vi "AK Befehl Auswerten.vi"(10 "Array":string[](array[string])) -> (2 "String für schreiben":string)   [LabVIEW 2020, in "AK-Schnittstelle.lvlib"]
uses:
  AK-Schnittstelle.lvlib
  Aktionen Stoernummern pruefen.ctl
  Aktionen Zustandsfehlerinformation.ctl
  Funktionstasten/Zustaende.ctl
  Funktionstasten/Funktionstasten.lvlib
  Funktionstasten/Betriebsart.ctl
  Funktionstasten/Funktionstasten-Aktion.ctl
  Aktionen Gespeicherte Werte.ctl
  Seiten/Log Konfig/LogKonfig.lvlib
  Seiten/Log Konfig/Aktionen Trigger.ctl
  Seiten/FT-IR/FT-IR.lvlib
  Seiten/FT-IR/FGV FT-IR Gasliste Aktionen.ctl
  Messdaten/Messdaten.lvlib
  Messdaten/Aktionen FGV Messdaten.ctl
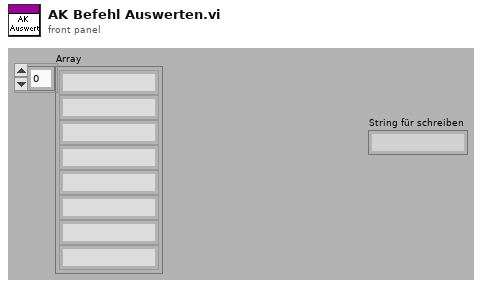
[diagram p1: front panel]
types:
  T1 = typedef "AK-Schnittstelle.lvlib/Aktionen Stoernummern pruefen.ctl" = enum16{"lesen", "prüfen"}
  T2 = typedef "AK-Schnittstelle.lvlib/Aktionen Zustandsfehlerinformation.ctl" = enum16{"OK", "Offline", "Busy", "Syntax Error", "Datenfehler"}
  T3 = typedef "AK-Schnittstelle.lvlib/Aktionen Gespeicherte Werte.ctl" = enum16{"lesen", "laden", "speichern", "Seriell", "TCP", "Diverse", "AKTIV", "AK-Namen"}
  T4 = typedef "Funktionstasten.lvlib/Funktionstasten-Aktion.ctl" = enum16{"Initialisieren", "Zustand setzen", "Taste gedrückt", "Fehler speichern", "Lesen", "Manuell", "Remote", "Bitparallel", "Samplepoint", "Zeit Prüfen", "reset Umschalten"}
  T5 = typedef "FT-IR.lvlib/FGV FT-IR Gasliste Aktionen.ctl" = enum16{"lesen", "Gasliste FT-IR", "Gasliste ausgelesen", "laden", "speichern", "löschen"}
  T6 = typedef "Messdaten.lvlib/Aktionen FGV Messdaten.ctl" = enum16{"lesen", "schreiben", "löschen", "Mittelwerte", "Komponente"}
  T7 = typedef "Funktionstasten.lvlib/Zustaende.ctl" = enum16{"Standby", "Pause", "Eco", "Messen", "Kalibrieren", "Spülen Filter", "Spülen Leitung", "Umgebungsluft", "0-Gas", "Cal-Gas", "CG zu PNS", "-------------", "Init 1", "Init 2", "Init 3", "Init 4", "Messen vorbereiten", "Messen durchführen", "Exit"}
  T8 = typedef "Funktionstasten.lvlib/Betriebsart.ctl" = enum16{"Manuell", "Remote", "Bitparallel"}
  T9 = typedef "LogKonfig.lvlib/Aktionen Trigger.ctl" = enum16{"lesen", "ALLE schreiben", "Trigger prüfen", "Trigger rücksetzen"}
  T10 = typedef "AK-Schnittstelle.lvlib/Diverse gespeicherte Werte.ctl" = cluster{"Kalibriergaseingang":i16, "SamplePoint":i16, "CalGas zu PNS":i16, "Gas-Reihenfolge":i16[], "Zeit 0-Gas":sgl, "Zeit CalGas":sgl, "AK Befehlssatz":T11}
  T11 = typedef "AK-Schnittstelle.lvlib/AK Befehlssatz.ctl" = enum16{"MEXA", "IAG v1.4", "AVL (Puma)", "PEUS"}
  T12 = typedef "LogKonfig.lvlib/Element Triggerereignisse.ctl" = cluster{"Trigger verwenden":T13, "Messwert":u16, "kl./gr.":u16, "Wert":sgl, "Puffergröße":sgl}
  T13 = typedef "LogKonfig.lvlib/Auswahlfeld aktiviert-deaktiviert.ctl" = u16
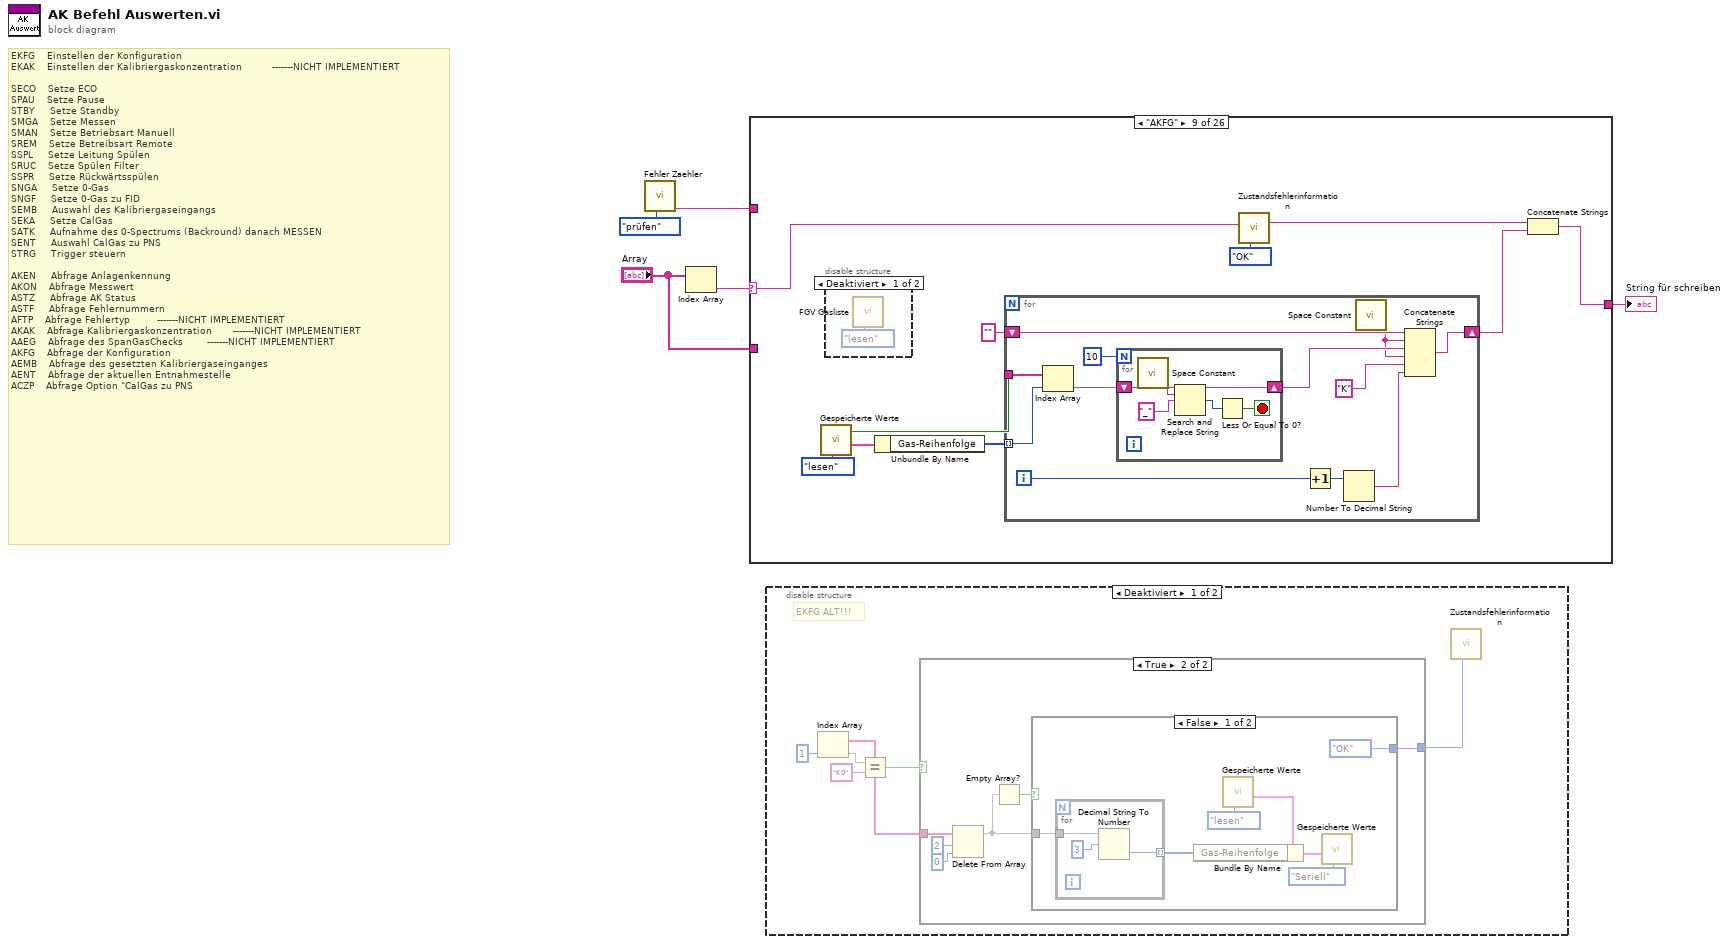
[diagram p0: block diagram]
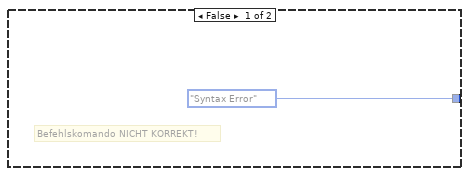
[diagram p2: hidden frame]
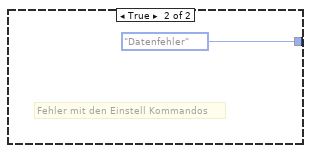
[diagram p3: hidden frame]
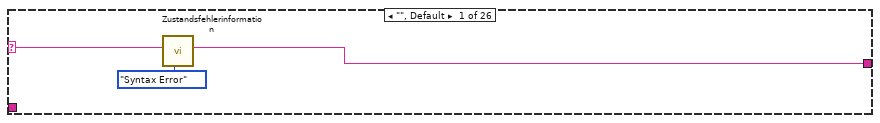
[diagram p5: hidden frame]
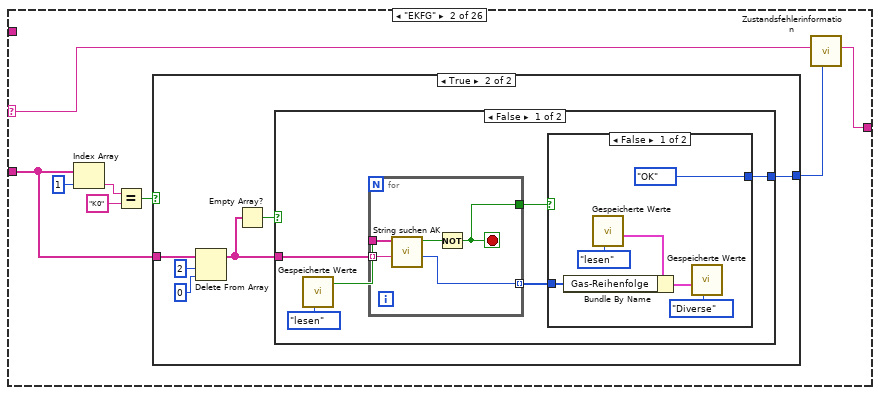
[diagram p6: hidden frame]
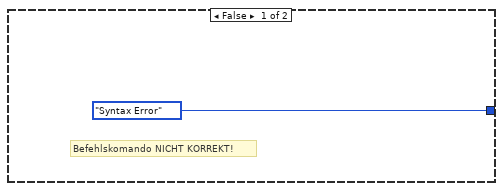
[diagram p7: hidden frame]
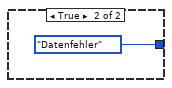
[diagram p8: hidden frame]
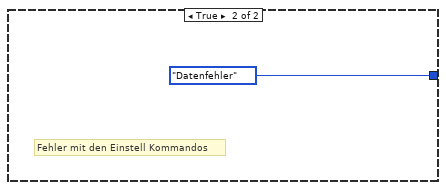
[diagram p9: hidden frame]
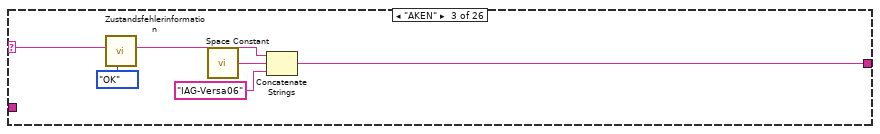
[diagram p10: hidden frame]
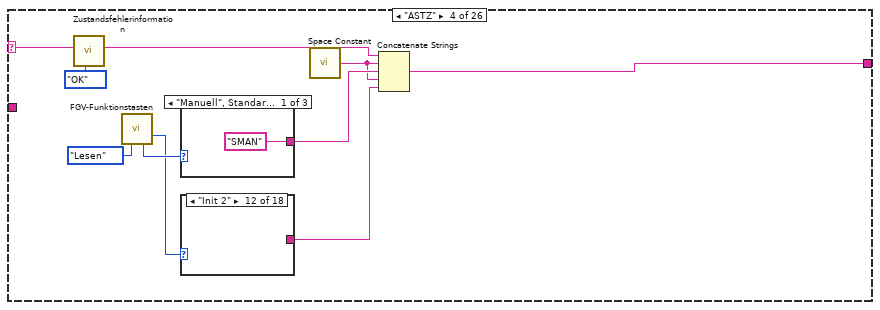
[diagram p11: hidden frame]
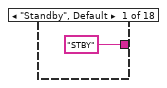
[diagram p12: hidden frame]
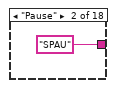
[diagram p13: hidden frame]
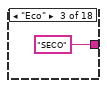
[diagram p14: hidden frame]
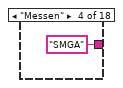
[diagram p15: hidden frame]
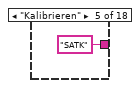
[diagram p16: hidden frame]
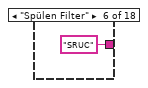
[diagram p17: hidden frame]
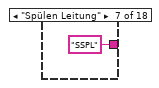
[diagram p18: hidden frame]
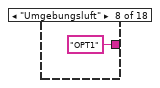
[diagram p19: hidden frame]
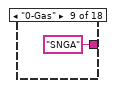
[diagram p20: hidden frame]
diagram:
  # "EKFG    Einstellen der Konfiguration\nEKAK    Einstellen der Kalibriergaskonzentration          -------NICHT IMPLEMENTIERT\n\nSECO    Setze ECO\nSPAU    Setze Pause\nSTBY     Setze Standby\nSMGA    Setze Messen\nSMAN    Setze Betriebsart Manuell\nSREM    Setze Betreibsart Remote\nSSPL     Setze Leitung Spülen\nSRUC    Setze Spülen Filter\nSSPR     Setze Rückwärtsspülen\nSNGA     Setze 0-Gas\nSNGF     Setze 0-Gas zu FID\nSEMB     Auswahl des Kalibriergaseingangs\nSEKA     Setze CalGas\nSATK     Aufnahme des 0-Spectrums (Backround) danach MESSEN\nSENT     Auswahl CalGas zu PNS\nSTRG     Trigger steuern\n\nAKEN     Abfrage Anlagenkennung\nAKON    Abfrage Messwert\nASTZ     Abfrage AK Status\nASTF     Abfrage Fehlernummern\nAFTP    Abfrage Fehlertyp         -------NICHT IMPLEMENTIERT\nAKAK    Abfrage Kalibriergaskonzentration       -------NICHT IMPLEMENTIERT\nAAEG    Abfrage des SpanGasChecks        -------NICHT IMPLEMENTIERT\nAKFG    Abfrage der Konfiguration\nAEMB    Abfrage des gesetzten Kalibriergaseinganges\nAENT    Abfrage der aktuellen Entnahmestelle\nACZP    Abfrage Option \"CalGas zu PNS"
  n1 = call "Fehler Zaehler.vi"("Aktionen"=Aktionen_Stoernummern_pruefen."prüfen") -> ("Fehlerzähler"=w3:string)  [unwired: 7 in, 3 out]
  n2 = Index Array(array="Array") -> (element=w2:string)  [unwired: 1 in]
  n3 = case shown="\"AKFG\"" w2 {
    selector: w2 -> [w7 w15 w45 w56 w76 w86 w95 w104 w114 w149 w194 w197 w200 w203 w206 w209 w213 w216 w220 w222 w235 w240 w261 w275 w279 w310]
    tunnel: [w6 w14 w47 w58 w78 w88 w97 w106 w116 w150 w193 w196 w199 w202 w205 w208 w212 w215 w219 w221 w234 w239 w260 w274 w278 w309] -> w5
    tunnel: w3 -> [_ _ _ _ _ _ _ _ _ _ _ _ _ _ _ _ _ _ _ _ _ _ _ _ _ _]
    tunnel: "Array" -> [_ w16 _ _ _ _ _ _ _ w140 _ _ _ _ _ _ _ _ _ _ _ w238 _ _ w277 w308]
    frame "", Default {
      n4 = call "Zustandsfehlerinformation.vi"("Aktionen"=Aktionen_Zustandsfehlerinformation."Syntax Error", "String"=w7) -> ("String"=w6:string)  [unwired: 9 in]
    }
    frame "EKFG" {
      n5 = Index Array(array=w16, index=1 ("Index")) -> (element=w12:string)
      n6 = Equal?(x=w12, y="K0") -> (x = y?=w10:bool)
      n7 = case shown="True" w10 {
        tunnel: w16 -> [_ w21]
        tunnel: [Aktionen_Zustandsfehlerinformation."Syntax Error" ("Aktionen") w18] -> w9
        frame False {
          # "Befehlskomando NICHT KORREKT!"
        }
        frame True {
          n8 = Delete From Array(array=w21, length=2 ("Länge"), index=0 ("Index")) -> (array with subset deleted=w20:string[])  [unwired: 1 out]
          n9 = Empty Array?(array=w20) -> (empty?=w19:bool)
          n10 = case shown="False" w19 {
            tunnel: w20 -> [w29 _]
            tunnel: [w25 Aktionen_Zustandsfehlerinformation."Datenfehler" ("Aktionen")] -> w18
            frame False {
              n11 = call "Gespeicherte Werte.vi"("Aktionen"=Aktionen_Gespeicherte_Werte."lesen") -> ("Port changed in"=w26:bool)  [unwired: 5 in, 5 out]
              n12 = for {
                tunnel: w29 -> [w32] mode=indexing
                tunnel: [w31] -> w28 mode=indexing
                tunnel: w26 -> [w33]
                tunnel: [w34] -> w24
                stop <- w34 stop-if-true
                n13 = call "String suchen AK.vi"("gesucht"=w32, "Namen"=w33) -> ("Index"=w31:i32, "Gefunden?"=w30:bool)  [unwired: 8 in]
                n14 = Not(x=w30) -> (.not. x?=w34:bool)
              }
              n15 = case shown="False" w24 {
                tunnel: w28 -> [w39 _]
                tunnel: [Aktionen_Zustandsfehlerinformation."OK" ("Aktionen") Aktionen_Zustandsfehlerinformation."Datenfehler" ("Aktionen")] -> w25
                frame False {
                  n16 = call "Gespeicherte Werte.vi"("Aktionen"=Aktionen_Gespeicherte_Werte."lesen") -> ("Diverse Werte"=w37:T10)  [unwired: 6 in, 4 out]
                  n17 = Bundle By Name(cluster=w37, "Gas-Reihenfolge"=w39) -> (w36:T10)
                  n18 = call "Gespeicherte Werte.vi"("Aktionen"=Aktionen_Gespeicherte_Werte."Diverse", "Diverse Werte"=w36) -> ()  [unwired: 5 in, 5 out]
                }
                frame True {
                }
              }
            }
            frame True {
              # "Fehler mit den Einstell Kommandos"
            }
          }
        }
      }
      n19 = call "Zustandsfehlerinformation.vi"("Aktionen"=w9, "String"=w15) -> ("String"=w14:string)  [unwired: 9 in]
    }
    frame "AKEN" {
      n20 = call "Zustandsfehlerinformation.vi"("Aktionen"=Aktionen_Zustandsfehlerinformation."OK", "String"=w45) -> ("String"=w44:string)  [unwired: 9 in]
      n21 = call <vilib>:"Space Constant.vi"() -> ("String"=w43:string)
      n22 = Concatenate Strings(w44, w43, "IAG-Versa06" ("String")) -> (w47:string)
    }
    frame "ASTZ" {
      n23 = call "Zustandsfehlerinformation.vi"("Aktionen"=Aktionen_Zustandsfehlerinformation."OK", "String"=w56) -> ("String"=w55:string)  [unwired: 9 in]
      n24 = call "FGV-Funktionstasten.vi"("Aktion"=Funktionstasten-Aktion."Lesen") -> ("ausgewählte Funktion"=w51:T7, "Betriebsart"=w53:T8)  [unwired: 7 in, 6 out]
      n25 = case shown="\"Manuell\", Standard" w53 {
        tunnel: ["SMAN" ("String") "SREM" ("String") "SBIT" ("String")] -> w52
        frame "Manuell", Default {
        }
        frame "Remote" {
        }
        frame "Bitparallel" {
        }
      }
      n26 = case shown="\"Init 2\"" w51 {
        tunnel: ["STBY" ("String") "SPAU" ("String") "SECO" ("String") "SMGA" ("String") "SATK" ("String") "SRUC" ("String") "SSPL" ("String") "OPT1" ("String") "SNGA" ("String") "OPT2" ("String") _ _ _ _ _ _ _ _] -> w49
        frame "Standby", Default {
        }
        frame "Pause" {
        }
        frame "Eco" {
        }
        frame "Messen" {
        }
        frame "Kalibrieren" {
        }
        frame "Spülen Filter" {
        }
        frame "Spülen Leitung" {
        }
        frame "Umgebungsluft" {
        }
        frame "0-Gas" {
        }
        frame "Cal-Gas" {
        }
        frame "Init 1" {
        }
        frame "Init 2" {
        }
        frame "-------------" {
        }
        frame "Init 3" {
        }
        frame "Init 4" {
        }
        frame "Messen vorbereiten" {
        }
        frame "Messen durchführen" {
        }
        frame "Exit" {
        }
      }
      n27 = call <vilib>:"Space Constant.vi"() -> ("String"=w50:string)
      n28 = Concatenate Strings(w55, w50, w52, w50, w49) -> (w58:string)
    }
    frame "ASTF" {
      n29 = call "Zustandsfehlerinformation.vi"("Aktionen"=Aktionen_Zustandsfehlerinformation."OK", "String"=w76) -> ("String"=w75:string)  [unwired: 9 in]
      n30 = call "Fehler Zaehler.vi"("Aktionen"=Aktionen_Stoernummern_pruefen."lesen") -> ("Fehler Nummern"=w73:string)  [unwired: 7 in, 3 out]
      n31 = call <vilib>:"Space Constant.vi"() -> ("String"=w72:string)
      n32 = Concatenate Strings(w75, w72, w73) -> (w78:string)
    }
    frame "AEMB" {
      n33 = call "Zustandsfehlerinformation.vi"("Aktionen"=Aktionen_Zustandsfehlerinformation."OK", "String"=w86) -> ("String"=w85:string)  [unwired: 9 in]
      n34 = call "Gespeicherte Werte.vi"("Aktionen"=Aktionen_Gespeicherte_Werte."lesen") -> ("Diverse Werte"=w79:T10)  [unwired: 6 in, 4 out]
      n35 = Unbundle By Name(w79) -> ("Kalibriergaseingang"=w83:i16)
      n36 = call <vilib>:"Space Constant.vi"() -> ("String"=w80:string)
      n37 = Number To Decimal String(number=w83) -> (decimal integer string=w81:string)  [unwired: 1 in]
      n38 = Concatenate Strings(w85, w80, "M" ("String"), w81) -> (w88:string)
    }
    frame "AENT" {
      n39 = call "Zustandsfehlerinformation.vi"("Aktionen"=Aktionen_Zustandsfehlerinformation."OK", "String"=w95) -> ("String"=w94:string)  [unwired: 9 in]
      n40 = call "FGV-Funktionstasten.vi"("Aktion"=Funktionstasten-Aktion."Lesen") -> ("Samplepoint"=w89:u16)  [unwired: 7 in, 7 out]
      n41 = call <vilib>:"Space Constant.vi"() -> ("String"=w91:string)
      n42 = Number To Decimal String(number=w89) -> (decimal integer string=w92:string)  [unwired: 1 in]
      n43 = Concatenate Strings(w94, w91, "M" ("String"), w92) -> (w97:string)
    }
    frame "ACZP" {
      n44 = call "Zustandsfehlerinformation.vi"("Aktionen"=Aktionen_Zustandsfehlerinformation."OK", "String"=w104) -> ("String"=w103:string)  [unwired: 9 in]
      n45 = call "Gespeicherte Werte.vi"("Aktionen"=Aktionen_Gespeicherte_Werte."lesen") -> ("Diverse Werte"=w98:T10)  [unwired: 6 in, 4 out]
      n46 = Unbundle By Name(w98) -> ("CalGas zu PNS"=w101:i16)
      n47 = call <vilib>:"Space Constant.vi"() -> ("String"=w99:string)
      n48 = Number To Decimal String(number=w101) -> (decimal integer string=w100:string)  [unwired: 1 in]
      n49 = Concatenate Strings(w103, w99, w100) -> (w106:string)
    }
    frame "AKFG" {
      n50 = call "Gespeicherte Werte.vi"("Aktionen"=Aktionen_Gespeicherte_Werte."lesen") -> ("Diverse Werte"=w109:T10, "Port changed in"=w107:bool)  [unwired: 5 in, 4 out]
      n51 = disable-structure shown="Deaktiviert" {
        frame Disabled {
          n52 = call "FGV Gasliste.vi"("Aktionen"=FGV_FT-IR_Gasliste_Aktionen."lesen") -> ()  [unwired: 8 in, 3 out]
        }
        frame Enabled {
        }
      }
      n53 = Unbundle By Name(w109) -> ("Gas-Reihenfolge"=w111:i16[])
      n54 = for {
        tunnel: w111 -> [w126] mode=indexing
        shift-right: [w129] -> w108
        shift-left: "" -> [w128]
        tunnel: w107 -> [w127]
        i -> [w119]
        n55 = Index Array(array=w127, index=w126) -> (element=w124)
        n56 = for {
          N: 10 -> [_]
          shift-right: [w134] -> w123
          shift-left: w124 -> [w135]
          stop <- w132 stop-if-true
          n57 = call <vilib>:"Space Constant.vi"() -> ("String"=w131:string)
          n58 = Search and Replace String(input string=w135, search string=w131, replace string="_") -> (result string=w134:string, number of replacements=w133:i32)  [unwired: 5 in, 2 out]
          n59 = Less Or Equal To 0?(x=w133) -> (x <= 0?=w132:bool)
        }
        n60 = Increment(x=w119) -> (x+1=w121:i32)
        n61 = Number To Decimal String(number=w121) -> (decimal integer string=w118:string)  [unwired: 1 in]
        n62 = call <vilib>:"Space Constant.vi"() -> ("String"=w122:string)
        n63 = Concatenate Strings(w128, w122, w123, w122, "K" ("String"), w118) -> (w129:string)
      }
      n64 = call "Zustandsfehlerinformation.vi"("Aktionen"=Aktionen_Zustandsfehlerinformation."OK", "String"=w114) -> ("String"=w113:string)  [unwired: 9 in]
      n65 = Concatenate Strings(w113, w108) -> (w116:string)
    }
    frame "AKON" {
      n66 = call "Gespeicherte Werte.vi"("Aktionen"=Aktionen_Gespeicherte_Werte."lesen") -> ("Diverse Werte"=w138:T10)  [unwired: 6 in, 4 out]
      n67 = Index Array(array=w140, index=1 ("Index")) -> (element=w143:string)
      n68 = Unbundle By Name(w138) -> ("Gas-Reihenfolge"=w146:i16[])
      n69 = Equal?(x=w143, y="K0") -> (x = y?=w141:bool)
      n70 = call "FGV Messdaten.vi"("Aktionen"=Aktionen_FGV_Messdaten."lesen") -> ("Aktuelle Messwerte"=w136:sgl[])  [unwired: 6 in, 8 out]
      n71 = case shown="False" w141 {
        tunnel: w146 -> [w153 w184]
        tunnel: [w151 w182] -> w145
        tunnel: w136 -> [w152 w181]
        tunnel: w140 -> [w157 _]
        tunnel: [w155 Aktionen_Zustandsfehlerinformation."OK" ("Aktionen")] -> w139
        frame False {
          n72 = Delete From Array(array=w157, length=1 ("Länge"), index=0 ("Index")) -> (array with subset deleted=w154:string[])  [unwired: 1 out]
          n73 = Empty Array?(array=w154) -> (empty?=w156:bool)
          n74 = case shown="False" w156 {
            tunnel: [Aktionen_Zustandsfehlerinformation."OK" ("Aktionen") Aktionen_Zustandsfehlerinformation."Datenfehler" ("Aktionen")] -> w155
            tunnel: w154 -> [w164 _]
            tunnel: w153 -> [w163 _]
            tunnel: w152 -> [w162 _]
            tunnel: [w161 ""] -> w151
            frame False {
              # "Je nach Abgefragten Kanal den RICHTIGEN\nMesswert heraussuchen!"
              n75 = for {
                tunnel: w164 -> [w177] mode=indexing
                tunnel: w163 -> [w175]
                tunnel: w162 -> [w174]
                shift-right: [w173] -> w161
                shift-left: "" -> [w170]
                n76 = Decimal String To Number(string=w177, offset=1 ("Offset (0)")) -> (number=w169:i32)  [unwired: 1 in, 1 out]
                n77 = Decrement(x=w169) -> (x-1=w168:i32)
                n78 = Index Array(array=w175, index=w168) -> (element=w166:i16)
                n79 = Index Array(array=w174, index=w166) -> (element=w172:sgl)
                n80 = call <vilib>:"Space Constant.vi"() -> ("String"=w167:string)
                n81 = Number To Fractional String(number=w172) -> (F-format string=w171:string)  [unwired: 3 in]
                n82 = Concatenate Strings(w170, w167, w171) -> (w173:string)
              }
            }
            frame True {
              # "Wenn der String leer ist, dann Datenfehler"
            }
          }
        }
        frame True {
          n83 = for {
            tunnel: w184 -> [w185] mode=indexing
            shift-right: [w191] -> w182
            shift-left: "" -> [w190]
            tunnel: w181 -> [w189]
            n84 = Index Array(array=w189, index=w185) -> (element=w188:sgl)
            n85 = Number To Fractional String(number=w188) -> (F-format string=w187:string)  [unwired: 3 in]
            n86 = call <vilib>:"Space Constant.vi"() -> ("String"=w186:string)
            n87 = Concatenate Strings(w190, w186, w187) -> (w191:string)
          }
        }
      }
      n88 = call "Zustandsfehlerinformation.vi"("Aktionen"=w139, "String"=w149) -> ("String"=w148:string)  [unwired: 9 in]
      n89 = Concatenate Strings(w148, w145) -> (w150:string)
    }
    frame "SECO" {
      n90 = call "Setze Zustand.vi"("AK Befehl"=w194, "Zustand"=Zustaende."Eco") -> ("Antwort String"=w193:string)  [unwired: 8 in, 1 out]
    }
    frame "SPAU" {
      n91 = call "Setze Zustand.vi"("AK Befehl"=w197, "Zustand"=Zustaende."Pause") -> ("Antwort String"=w196:string)  [unwired: 8 in, 1 out]
    }
    frame "STBY" {
      n92 = call "Setze Zustand.vi"("AK Befehl"=w200, "Zustand"=Zustaende."Standby") -> ("Antwort String"=w199:string)  [unwired: 8 in, 1 out]
    }
    frame "SMGA" {
      n93 = call "Setze Zustand.vi"("AK Befehl"=w203, "Zustand"=Zustaende."Messen") -> ("Antwort String"=w202:string)  [unwired: 8 in, 1 out]
    }
    frame "SSPL" {
      n94 = call "Setze Zustand.vi"("AK Befehl"=w206, "Zustand"=Zustaende."Spülen Leitung") -> ("Antwort String"=w205:string)  [unwired: 8 in, 1 out]
    }
    frame "SRUC" {
      n95 = call "Setze Zustand.vi"("AK Befehl"=w209, "Zustand"=Zustaende."Spülen Filter") -> ("Antwort String"=w208:string)  [unwired: 8 in, 1 out]
    }
    frame "SSPR" {
      n96 = call "Setze Zustand.vi"("Befehl nicht vorhanden!"=TRUE, "AK Befehl"=w213, "Zustand"=Zustaende."Standby") -> ("Antwort String"=w212:string)  [unwired: 7 in, 1 out]
    }
    frame "SNGA" {
      n97 = call "Setze Zustand.vi"("AK Befehl"=w216, "Zustand"=Zustaende."0-Gas") -> ("Antwort String"=w215:string)  [unwired: 8 in, 1 out]
    }
    frame "SNGF" {
      n98 = call "Setze Zustand.vi"("Befehl nicht vorhanden!"=TRUE, "AK Befehl"=w220, "Zustand"=Zustaende."Standby") -> ("Antwort String"=w219:string)  [unwired: 7 in, 1 out]
    }
    frame "SMAN" {
      n99 = call "FGV-Funktionstasten.vi"("Aktion"=Funktionstasten-Aktion."Lesen") -> ("Betriebsart"=w226:T8)  [unwired: 7 in, 7 out]
      n100 = Equal?(x=w226, y=Betriebsart."Remote" ("Betriebsart")) -> (x = y?=w223:bool)
      n101 = case shown="True" w223 {
        tunnel: w222 -> [w229 w232]
        tunnel: [w227 w231] -> w221
        frame False {
          n102 = call "Zustandsfehlerinformation.vi"("Aktionen"=Aktionen_Zustandsfehlerinformation."Offline", "String"=w229) -> ("String"=w227:string)  [unwired: 9 in]
        }
        frame True {
          n103 = call "Zustandsfehlerinformation.vi"("Aktionen"=Aktionen_Zustandsfehlerinformation."OK", "String"=w232) -> ("String"=w231:string)  [unwired: 9 in]
          n104 = call "FGV-Funktionstasten.vi"("Aktion"=Funktionstasten-Aktion."Manuell") -> ()  [unwired: 7 in, 8 out]
        }
      }
    }
    frame "SREM" {
      n105 = call "Zustandsfehlerinformation.vi"("Aktionen"=Aktionen_Zustandsfehlerinformation."OK", "String"=w235) -> ("String"=w234:string)  [unwired: 9 in]
      n106 = call "FGV-Funktionstasten.vi"("Aktion"=Funktionstasten-Aktion."Remote") -> ()  [unwired: 7 in, 8 out]
    }
    frame "SEMB" {
      n107 = call "FGV-Funktionstasten.vi"("Aktion"=Funktionstasten-Aktion."Lesen") -> ("Betriebsart"=w243:T8)  [unwired: 7 in, 7 out]
      n108 = Equal?(x=w243, y=Betriebsart."Remote" ("Betriebsart")) -> (x = y?=w244:bool)
      n109 = case shown="True" w244 {
        tunnel: w240 -> [w246 w258]
        tunnel: [w245 w257] -> w239
        tunnel: w238 -> [_ w256]
        frame False {
          n110 = call "Zustandsfehlerinformation.vi"("Aktionen"=Aktionen_Zustandsfehlerinformation."Offline", "String"=w246) -> ("String"=w245:string)  [unwired: 9 in]
        }
        frame True {
          n111 = Index Array(array=w256, index=2 ("Index")) -> (element=w254:string)
          n112 = call "Zustandsfehlerinformation.vi"("Aktionen"=Aktionen_Zustandsfehlerinformation."OK", "String"=w258) -> ("String"=w257:string)  [unwired: 9 in]
          n113 = Decimal String To Number(string=w254, offset=1 ("Offset (0)")) -> (number=w250:i32)  [unwired: 1 in, 1 out]
          n114 = call "Gespeicherte Werte.vi"("Aktionen"=Aktionen_Gespeicherte_Werte."lesen") -> ("Diverse Werte"=w249:T10)  [unwired: 6 in, 4 out]
          n115 = Bundle By Name(cluster=w249, "Kalibriergaseingang"=w250) -> (w248:T10)
          n116 = call "Gespeicherte Werte.vi"("Aktionen"=Aktionen_Gespeicherte_Werte."Seriell", "Diverse Werte"=w248) -> ()  [unwired: 5 in, 5 out]
        }
      }
    }
    frame "SEKA" {
      n117 = call "FGV-Funktionstasten.vi"("Aktion"=Funktionstasten-Aktion."Lesen") -> ("Betriebsart"=w264:T8)  [unwired: 7 in, 7 out]
      n118 = Equal?(x=w264, y=Betriebsart."Remote" ("Betriebsart")) -> (x = y?=w265:bool)
      n119 = case shown="True" w265 {
        tunnel: w261 -> [w267 w270]
        tunnel: [w266 w269] -> w260
        frame False {
          n120 = call "Zustandsfehlerinformation.vi"("Aktionen"=Aktionen_Zustandsfehlerinformation."Offline", "String"=w267) -> ("String"=w266:string)  [unwired: 9 in]
        }
        frame True {
          n121 = disable-structure shown="Deaktiviert" {
            frame Disabled {
              n122 = call "Gespeicherte Werte.vi"("Aktionen"=Aktionen_Gespeicherte_Werte."lesen") -> ("Diverse Werte"=w272:T10)  [unwired: 6 in, 4 out]
              n123 = Unbundle By Name(w272) -> ()  [unwired: 1 out]
            }
            frame Enabled {
            }
          }
          n124 = call "Zustandsfehlerinformation.vi"("Aktionen"=Aktionen_Zustandsfehlerinformation."OK", "String"=w270) -> ("String"=w269:string)  [unwired: 9 in]
        }
      }
    }
    frame "SATK" {
      n125 = call "Setze Zustand.vi"("AK Befehl"=w275, "Zustand"=Zustaende."Kalibrieren") -> ("Antwort String"=w274:string)  [unwired: 8 in, 1 out]
    }
    frame "SENT" {
      n126 = call "FGV-Funktionstasten.vi"("Aktion"=Funktionstasten-Aktion."Lesen") -> ("Betriebsart"=w282:T8)  [unwired: 7 in, 7 out]
      n127 = Equal?(x=w282, y=Betriebsart."Remote" ("Betriebsart")) -> (x = y?=w283:bool)
      n128 = case shown="True" w283 {
        tunnel: w279 -> [w285 w301]
        tunnel: [w284 w300] -> w278
        tunnel: w277 -> [_ w299]
        frame False {
          n129 = call "Zustandsfehlerinformation.vi"("Aktionen"=Aktionen_Zustandsfehlerinformation."Offline", "String"=w285) -> ("String"=w284:string)  [unwired: 9 in]
        }
        frame True {
          n130 = Index Array(array=w299, index #1=2 ("Index"), index #2=3 ("Index")) -> (element #1=w297:string, element #2=w293:string)
          n131 = call "Zustandsfehlerinformation.vi"("Aktionen"=Aktionen_Zustandsfehlerinformation."OK", "String"=w301) -> ("String"=w300:string)  [unwired: 9 in]
          n132 = Empty String/Path?(string/path=w293) -> (empty?=w295:bool)
          n133 = case shown="True" w295 {
            tunnel: [w303 w306] -> w291
            tunnel: w293 -> [w304 _]
            frame False {
              n134 = Decimal String To Number(string=w304) -> (number=w303:i32)  [unwired: 2 in, 1 out]
            }
            frame True {
              n135 = call "Gespeicherte Werte.vi"("Aktionen"=Aktionen_Gespeicherte_Werte."lesen") -> ("Diverse Werte"=w305:T10)  [unwired: 6 in, 4 out]
              n136 = Unbundle By Name(w305) -> ("CalGas zu PNS"=w306:i16)
            }
          }
          n137 = Decimal String To Number(string=w297) -> (number=w287:i32)  [unwired: 2 in, 1 out]
          n138 = call "FGV-Funktionstasten.vi"("Samplepoint"=w287, "Aktion"=Funktionstasten-Aktion."Samplepoint") -> ()  [unwired: 6 in, 8 out]
          n139 = call "Gespeicherte Werte.vi"("Aktionen"=Aktionen_Gespeicherte_Werte."lesen") -> ("Diverse Werte"=w290:T10)  [unwired: 6 in, 4 out]
          n140 = Bundle By Name(cluster=w290, "SamplePoint"=w287, "CalGas zu PNS"=w291) -> (w289:T10)
          n141 = call "Gespeicherte Werte.vi"("Aktionen"=Aktionen_Gespeicherte_Werte."Seriell", "Diverse Werte"=w289) -> ()  [unwired: 5 in, 5 out]
        }
      }
    }
    frame "STRG" {
      n142 = call "FGV-Funktionstasten.vi"("Aktion"=Funktionstasten-Aktion."Lesen") -> ("Betriebsart"=w313:T8)  [unwired: 7 in, 7 out]
      n143 = Equal?(x=w313, y=Betriebsart."Remote" ("Betriebsart")) -> (x = y?=w314:bool)
      n144 = case shown="True" w314 {
        tunnel: w310 -> [w316 w323]
        tunnel: [w315 w322] -> w309
        tunnel: w308 -> [_ w321]
        frame False {
          n145 = call "Zustandsfehlerinformation.vi"("Aktionen"=Aktionen_Zustandsfehlerinformation."Offline", "String"=w316) -> ("String"=w315:string)  [unwired: 9 in]
        }
        frame True {
          n146 = Index Array(array=w321, index=2 ("Index")) -> (element=w319:string)
          n147 = call "Zustandsfehlerinformation.vi"("Aktionen"=Aktionen_Zustandsfehlerinformation."OK", "String"=w323) -> ("String"=w322:string)  [unwired: 9 in]
          n148 = Empty String/Path?(string/path=w319) -> (empty?=w318:bool)
          n149 = case shown="False" w318 {
            tunnel: w319 -> [w330 _]
            frame False {
              n150 = Decimal String To Number(string=w330) -> (number=w327:i32)  [unwired: 2 in, 1 out]
              n151 = call "FGV Trigger.vi"("Aktion"=Aktionen_Trigger."lesen") -> ("Triggerereignis neu"=w326:T12)  [unwired: 7 in, 3 out]
              n152 = Bundle By Name(cluster=w326, "Trigger verwenden"=w327) -> (w325:T12)
              n153 = call "FGV Trigger.vi"("Aktion"=Aktionen_Trigger."ALLE schreiben", "Triggerereignis"=w325) -> ()  [unwired: 6 in, 4 out]
            }
            frame True {
            }
          }
        }
      }
    }
  }
  "String für schreiben" <- w5
  n154 = disable-structure shown="Deaktiviert" {
    frame Disabled {
      # "EKFG ALT!!!"
      n155 = Index Array(array=w334, index=1 ("Index")) -> (element=w337)
      n156 = Equal?(x=w337, y="K0") -> (x = y?=w335:bool)
      n157 = case shown="True" w335 {
        tunnel: [_ w343] -> w334
        tunnel: [Aktionen_Zustandsfehlerinformation."Syntax Error" ("Aktionen") w340] -> w332
        frame False {
          # "Befehlskomando NICHT KORREKT!"
        }
        frame True {
          n158 = Delete From Array(array=w343, length=2 ("Länge"), index=0 ("Index")) -> (array with subset deleted=w342)  [unwired: 1 out]
          n159 = Empty Array?(array=w342) -> (empty?=w341:bool)
          n160 = case shown="False" w341 {
            tunnel: w342 -> [w352 _]
            tunnel: [Aktionen_Zustandsfehlerinformation."OK" ("Aktionen") Aktionen_Zustandsfehlerinformation."Datenfehler" ("Aktionen")] -> w340
            frame False {
              n161 = for {
                tunnel: w352 -> [w354]
                tunnel: [w353] -> w350 mode=indexing
                n162 = Decimal String To Number(string=w354, offset=3 ("Offset (0)")) -> (number=w353:i32)  [unwired: 1 in, 1 out]
              }
              n163 = call "Gespeicherte Werte.vi"("Aktionen"=Aktionen_Gespeicherte_Werte."lesen") -> ("Diverse Werte"=w347:T10)  [unwired: 6 in, 4 out]
              n164 = Bundle By Name(cluster=w347, "Gas-Reihenfolge"=w350) -> (w346:T10)
              n165 = call "Gespeicherte Werte.vi"("Aktionen"=Aktionen_Gespeicherte_Werte."Seriell", "Diverse Werte"=w346) -> ()  [unwired: 5 in, 5 out]
            }
            frame True {
              # "Fehler mit den Einstell Kommandos"
            }
          }
        }
      }
      n166 = call "Zustandsfehlerinformation.vi"("Aktionen"=w332) -> (2:"String"=w331:string, 10:"String"=w333:string)  [unwired: 9 in]
    }
    frame Enabled {
    }
  }
